vi "F Dwf Enum Device Type.vi"(8 "error in (no error)":errorcluster, 9 "pDeviceRevision":i32, 10 "pDeviceId":i32, 11 "idxDevice":i32) -> (0 "error out":errorcluster, 1 "pDeviceRevision out":i32, 2 "pDeviceId out":i32, 3 "function return":i32)   [LabVIEW 2021, in "Olasdwf.lvlib"]
doc: "DWFAPI int FDwfEnumDeviceType(int idxDevice, DEVID *pDeviceId, DEVVER *pDeviceRevision);"
uses:
  Olasdwf.lvlib
  Windows/System32/dwf.dll
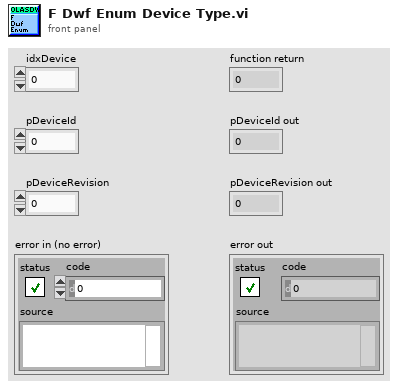
[diagram p1: front panel]
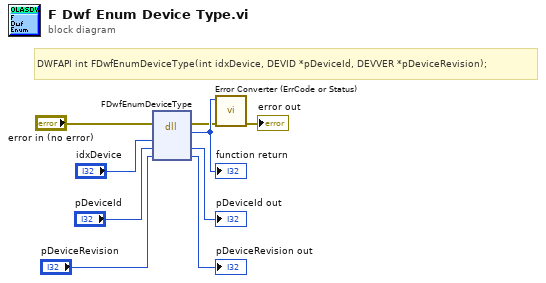
[diagram p0: block diagram]
diagram:
  # "DWFAPI int FDwfEnumDeviceType(int idxDevice, DEVID *pDeviceId, DEVVER *pDeviceRevision);"
  n1 = dll-call lib="/Windows/System32/dwf.*" fn="FDwfEnumDeviceType"(error in="error in (no error)", "idxDevice"="idxDevice", "pDeviceId"="pDeviceId", "pDeviceRevision"="pDeviceRevision") -> (error out=w2:errorcluster, w9:i32, "pDeviceId"=→"pDeviceId out":i32, "pDeviceRevision"=→"pDeviceRevision out":i32)  [unwired: 3 in, 1 out]
  "function return" <- w9
  n2 = call "Error Converter (ErrCode or Status).vi"("error in (no error)"=w2, "error code"=w9) -> ("error out"=→"error out":errorcluster)  [unwired: 9 in]
